vi "Endpoint-Default Config.vi"() -> (0 "Default Endpoint Config":T1[](array[typedef])=[{"Name"="Right", "Modality"=enum."Unspecified", "Laterality"=enum."N/A", "CalFile"=path "", "Audiogram"=path "", "reuse cal?"=FALSE}, {"Name"="Left", "Modality"=enum."Unspecified", "Laterality"=enum."N/A", "CalFile"=path "", "Audiogram"=path "", "reuse cal?"=FALSE}])   [LabVIEW 2020]
uses:
  Endpoint-Spec.ctl
  Endpoint-Modality.ctl
  Endpoint-Laterality.ctl
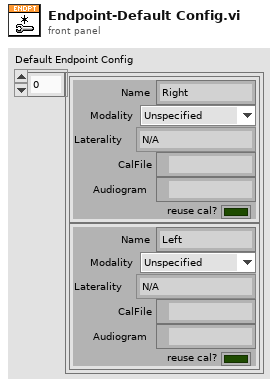
[diagram p1: front panel]
types:
  T1 = typedef "Endpoint-Spec.ctl" = cluster{"Name":string, "Modality":T2, "Laterality":T3, "CalFile":path, "Audiogram":path, "reuse cal?":bool}
  T2 = typedef "Endpoint-Modality.ctl" = enum16{"Unspecified", "Acoustic", "Electric", "Optical"}
  T3 = typedef "Endpoint-Laterality.ctl" = enum16{"N/A", "Right", "Left"}
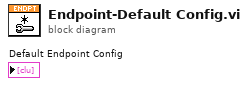
[diagram p0: block diagram]
diagram:
